vi "Write debugLevel.vi"(8 "error in (no error)":errorcluster, 10 "debugLevel":T1, 11 "TCSDebug in":refnum<class "TCSDebug.lvclass">) -> (0 "error out":errorcluster, 3 "TCSDebug out":refnum<class "TCSDebug.lvclass">)   [LabVIEW 2022 SP3, in "TCSDataDefinitions.lvlib" / "TCSCommand.lvlib" / "TCSDebug.lvclass"]
uses:
  TCSDebug.lvclass
  Enumerations/TCSDebuLevelTypes.ctl
  TCSDebug.lvclass/TCSDebug.ctl
  TCSCommand.lvlib
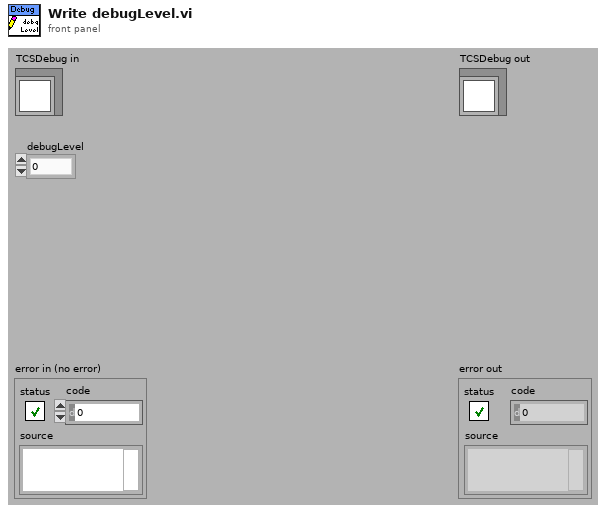
[diagram p1: front panel]
types:
  T1 = typedef "TCSDataDefinitions.lvlib/TCSCommand.lvlib/TCSDebuLevelTypes.ctl" = enum16{"0", "1", "2", "3", "4", "5", "6", "7", "8", "9", "10"}
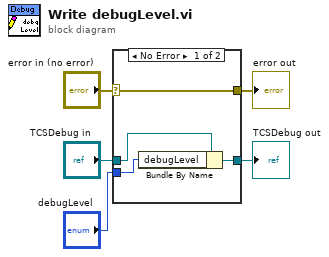
[diagram p0: block diagram]
diagram:
  n1 = case shown="No Error" "error in (no error)" {
    selector: "error in (no error)" -> [w9 w10]
    tunnel: [w9 w10] -> w4
    tunnel: [w7 w11] -> w2
    tunnel: "TCSDebug in" -> [w8 w11]
    tunnel: "debugLevel" -> [w6 _]
    frame No Error {
      n2 = Bundle By Name(cluster=w8, "debugLevel"=w6) -> (w7:refnum<class "TCSDebug.lvclass">)
    }
    frame Error {
    }
  }
  "error out" <- w4
  "TCSDebug out" <- w2
